vi "Hochdruckregler_PID.vi"(0 "Regler Hochdruck":bool, 2 "Steuereingang":dbl, 9 "Solldruck":dbl format="%.2f", 12 "PI05":dbl[](array[numeric]), 13 "Exp.V":dbl, 14 "reinitialize? (F) in":bool) -> (4 "Expansionsstellung":dbl, 6 "änderung expansion":dbl format="%.2f", 8 "upper limit out":dbl)   [LabVIEW 2015]
uses:
  <vilib>/addons/control/pid/pid.llb/PID (DBL).vi
  <vilib>/addons/control/pid/NI_PID_pid.lvlib
panel:
  in  "Hochdrucksteuerung":bool
  in  "lower limit":dbl=10.0
  in  "upper limit":dbl=100.0
  in  "PID gains":T1={"proportional gain (Kc)"=2.61, "integral time (Ti, min)"=1.0, "derivative time (Td, min)"=0.0} {"derivative time (Td, min)" format="%.3f"; "integral time (Ti, min)" format="%.3f"; "proportional gain (Kc)" format="%.3f"}
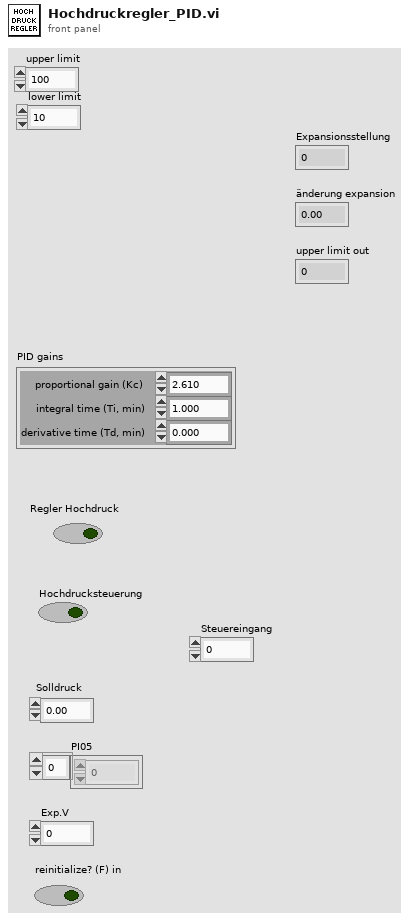
[diagram p1: front panel]
types:
  T1 = cluster{"proportional gain (Kc)":dbl, "integral time (Ti, min)":dbl, "derivative time (Td, min)":dbl}
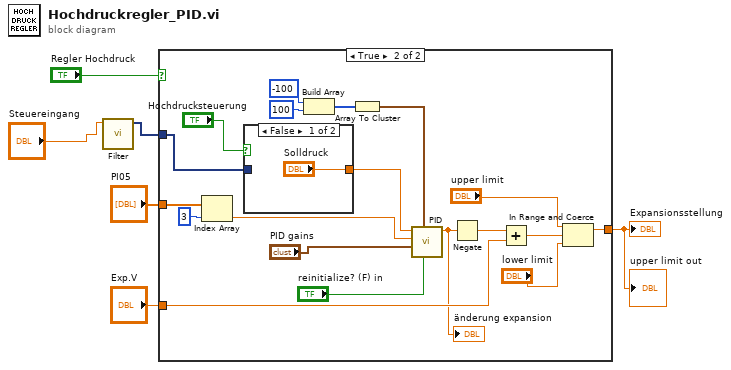
[diagram p0: block diagram]
diagram:
  n1 = call "Filter"("Signal"="Steuereingang") -> ("Filtered Signal"=w1:dynamicdata)  [unwired: 9 in, 1 out]
  n2 = case shown="True" "Regler Hochdruck" {
    tunnel: "PI05" -> [_ w25]
    tunnel: "Exp.V" -> [w7 w17]
    tunnel: [w7 w16] -> w5
    tunnel: w1 -> [_ w12]
    frame False {
    }
    frame True {
      n3 = Index Array(array=w25, index=3) -> (element=w19:dbl)
      n4 = case shown="False" "Hochdrucksteuerung" {
        tunnel: ["Solldruck" w28] -> w18
        tunnel: w12 -> [_ w28]
        frame False {
        }
        frame True {
        }
      }
      n5 = Build Array(-100, 100) -> (w23:i32[])
      n6 = Array To Cluster(array=w23) -> (cluster=w20:cluster{"[0]":i32, "[1]":i32})
      n7 = call-poly <vilib>:"PID.vi"("reinitialize? (F)"="reinitialize? (F) in", "output range"=w20, "PID gains"="PID gains", "process variable"=w19, "setpoint"=w18) -> ("output"=w13:dbl)  [unwired: 5 in, 1 out]
      "änderung expansion" <- w13
      n8 = Negate(x=w13) -> (-x=w14:dbl)
      n9 = Add(x=w14, y=w17) -> (x+y=w15:dbl)
      n10 = In Range and Coerce(upper limit="upper limit", x=w15, lower limit="lower limit") -> (coerced(x)=w16:dbl)  [unwired: 1 out]
    }
  }
  "Expansionsstellung" <- w5
  "upper limit out" <- w5
